vi "MB Get Device Info.vi"(8 "error in (no error)":errorcluster, 11 "TCP Ref:ValBlock":refnum<k5>) -> (0 "error out":errorcluster, 1 "MFC Info":T1, 3 "dup TCP Ref:ValBlock":refnum<k5>)   [LabVIEW 2011]
doc: "This VI reads the device identification of an MKS Modbus MFC. It reads all 9 object ID's and returns them in a cluster."
uses:
  EtherNet.lib/Modbus/mb Ethernet.llb/MB Modbus Data Unit.ctl
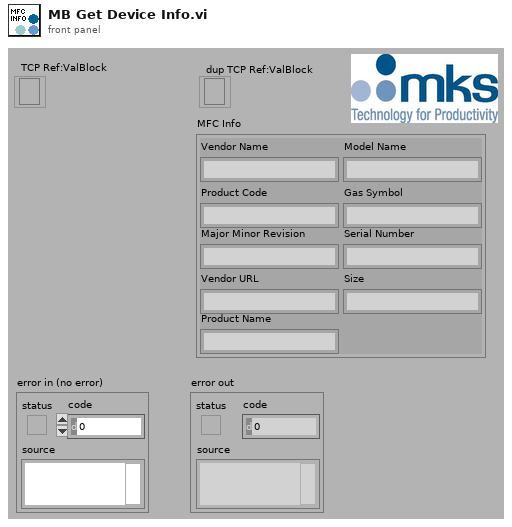
[diagram p1: front panel]
types:
  T1 = cluster{"Vendor Name":string, "Product Code":string, "Major Minor Revision":string, "Vendor URL":string, "Product Name":string, "Model Name":string, "Gas Symbol":string, "Serial Number":string, "Size":string}
  T2 = typedef "MB Modbus Data Unit.ctl" = cluster{"Function Code":u8, "Data":u8[]}
  T3 = cluster{"[0]":string, "[1]":string, "[2]":string, "[3]":string, "[4]":string, "[5]":string, "[6]":string, "[7]":string, "[8]":string}
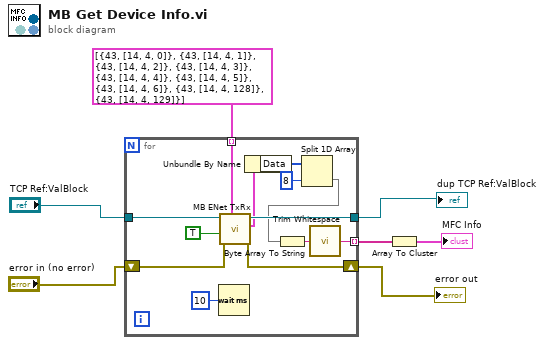
[diagram p0: block diagram]
diagram:
  n1 = for {
    shift-right: [w19] -> w4
    shift-left: "error in (no error)" -> [w20]
    tunnel: T2[] [{"Function Code"=43, "Data"=[14, 4, 0]}, {"Function Code"=43, "Data"=[14, 4, 1]}, {"Function Code"=43, "Data"=[14, 4, 2]}, {"Function Code"=43, "Data"=[14, 4, 3]}, {"Function Code"=43, "Data"=[14, 4, 4]}, {"Function Code"=43, "Data"=[14, 4, 5]}, {"Function Code"=43, "Data"=[14, 4, 6]}, {"Function Code"=43, "Data"=[14, 4, 128]}, {"Function Code"=43, "Data"=[14, 4, 129]}] -> [w18] mode=indexing
    tunnel: "TCP Ref:ValBlock" -> [w16]
    tunnel: [w15] -> w5
    tunnel: [w14] -> w3 mode=indexing
    n2 = Wait (ms)(milliseconds to wait=u32 10) -> ()  [unwired: 1 out]
    n3 = call "MB ENet TxRx.vi"("Modbus Data Unit In"=w18, "error in (no error)"=w20, "Use MODBUS Data Unit?"=TRUE, "TCP Ref:ValBlock"=w16) -> ("error out"=w19:errorcluster, "Modbus Data Unit Out"=w8:T2, "dup TCP Ref:ValBlock"=w15:refnum<k5>)  [unwired: 3 in, 2 out]
    n4 = Unbundle By Name(w8) -> ("Data"=w11:u8[])
    n5 = Split 1D Array(array=w11, index=8) -> (second subarray=w9:u8[])  [unwired: 1 out]
    n6 = Byte Array To String(unsigned byte array=w9) -> (string=w12:string)
    n7 = call <vilib>:"Trim Whitespace.vi"("string"=w12) -> ("trimmed string"=w14:string)  [unwired: 1 in]
  }
  "error out" <- w4
  "dup TCP Ref:ValBlock" <- w5
  n8 = Array To Cluster(array=w3) -> (cluster=→"MFC Info":T3)
